vi "SetTiles.vi"(8 "error in (no error)":errorcluster, 9 "Position":T1, 10 "TileCodes":u32[][](array[numeric])) -> (0 "error out":errorcluster)   [LabVIEW 2019, in "RT_Game.lvlib" / "Engine.lvclass"]
uses:
  Engine.lvclass
  Coordinate.ctl
  SetTilesData.ctl
  MessageCluster.ctl
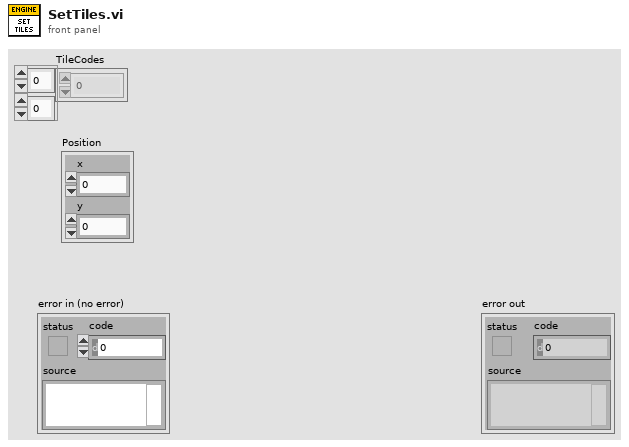
[diagram p1: front panel]
types:
  T1 = typedef "RT_Game.lvlib/Engine.lvclass/Coordinate.ctl" = cluster{"x":dbl, "y":dbl}
  T2 = typedef "RT_Game.lvlib/Engine.lvclass/MessageCluster.ctl" = cluster{"Message":string, "Data":variant}
  T3 = typedef "RT_Game.lvlib/Engine.lvclass/SetTilesData.ctl" = cluster{"TileCodes":u32[][], "Position":T1}
  T4 = typedef "RT_Game.lvlib/Engine.lvclass/Queues.ctl" = cluster{"MusicQueue":refnum<queue>, "TilesQueue":refnum<queue>, "SoundsQueue":refnum<queue>}
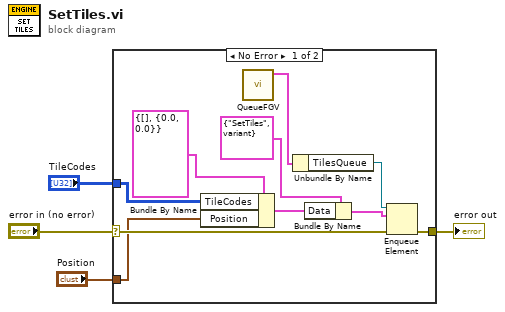
[diagram p0: block diagram]
diagram:
  n1 = case shown="No Error" "error in (no error)" {
    selector: "error in (no error)" -> [w14 w15]
    tunnel: [w13 w15] -> w3
    tunnel: "Position" -> [w8 _]
    tunnel: "TileCodes" -> [w7 _]
    frame No Error {
      n2 = Bundle By Name(cluster=T3 {"TileCodes"=[], "Position"={"x"=0.0, "y"=0.0}} ("SetTilesData"), "TileCodes"=w7, "Position"=w8) -> (w9:T3)
      n3 = call "QueueFGV.vi"() -> ("Queues out"=w6:T4)  [unwired: 10 in, 1 out]
      n4 = Unbundle By Name(w6) -> ("TilesQueue"=w5:refnum<queue>)
      n5 = Bundle By Name(cluster=T2 {"Message"="SetTiles", "Data"=variant} ("element"), "Data"=w9) -> (w11:T2)
      n6 = Enqueue Element(queue=w5, element=w11, error in (no error)=w14) -> (error out=w13:errorcluster)  [unwired: 1 in, 2 out]
    }
    frame Error {
    }
  }
  "error out" <- w3
